vi "AMZ_S3_APIHLP_Parse Set Versioning Request Parameters.vi"(6 "Auth device data":T2, 7 "error in (no error)":errorcluster, 10 "VersioningConfiguration":T3) -> (0 "error out":errorcluster, 3 "HTTP Headers":T1[](array[typedef]), 4 "PUT Data":string)   [LabVIEW 2015, in "LV Interface for Amazon S3.lvlib"]
uses:
  LV Interface for Amazon S3.lvlib
  Typedefs/AMZ_S3_API_VersioningConfiguration.ctl
  Typedefs/AMZ_S3_Versioning Status.ctl
  Typedefs/AMZ_S3_MFA Delete.ctl
  Typedefs/AMZ_S3_Auth Device Data.ctl
  Typedefs/AMZ_S3_HTTP Header-Value pair.ctl
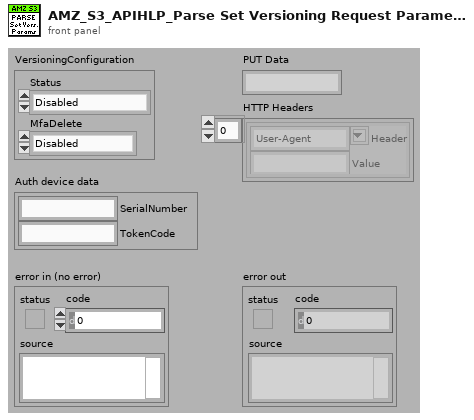
[diagram p1: front panel]
types:
  T1 = typedef "LV Interface for Amazon S3.lvlib/AMZ_S3_HTTP Header-Value pair.ctl" = cluster{"Header":string, "Value":string}
  T2 = typedef "LV Interface for Amazon S3.lvlib/AMZ_S3_Auth Device Data.ctl" = cluster{"SerialNumber":string, "TokenCode":string}
  T3 = typedef "LV Interface for Amazon S3.lvlib/AMZ_S3_API_VersioningConfiguration.ctl" = cluster{"Status":T4, "MfaDelete":T5}
  T4 = typedef "LV Interface for Amazon S3.lvlib/AMZ_S3_Versioning Status.ctl" = enum16{"Disabled", "Suspended", "Enabled"}
  T5 = typedef "LV Interface for Amazon S3.lvlib/AMZ_S3_MFA Delete.ctl" = enum16{"Disabled", "Enabled"}
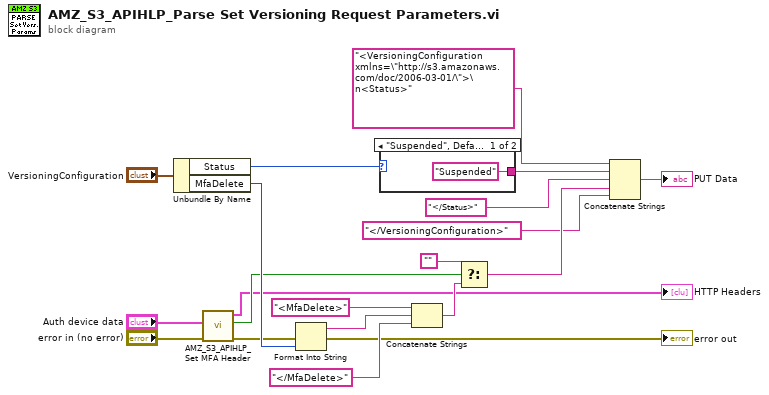
[diagram p0: block diagram]
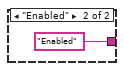
[diagram p2: hidden frame]
diagram:
  n1 = Unbundle By Name("VersioningConfiguration") -> ("Status"=w20:T4, "MfaDelete"=w7:T5)
  n2 = call "AMZ_S3_APIHLP_Set MFA Header.vi"("error in (no error)"="error in (no error)", "Auth device data"="Auth device data") -> ("error out"=w3:errorcluster, "Header set?"=w2:bool, "HTTP Headers"=→"HTTP Headers":T1[])  [unwired: 7 in]
  n3 = Format Into String(error in=w3, w7) -> (resulting string=w6:string, error out=→"error out":errorcluster)  [unwired: 2 in]
  n4 = case shown="\"Suspended\", Default" w20 {
    tunnel: ["Suspended" "Enabled"] -> w14
    frame "Suspended", Default {
    }
    frame "Enabled" {
    }
  }
  n5 = Concatenate Strings("<MfaDelete>", w6, "</MfaDelete>") -> (w15:string)
  n6 = Select(t="", s=w2, f=w15) -> (s? t:f=w11:string)
  n7 = Concatenate Strings("<VersioningConfiguration xmlns=\"http://s3.amazonaws.com/doc/2006-03-01/\">\n<Status>", w14, "</Status>", w11, "</VersioningConfiguration>") -> (→"PUT Data":string)
